vi "State Machine.vi"() -> ()   [LabVIEW 2014]
uses:
  Enum.ctl
panel:
  in  "STOP":bool
  in  "Executer le processus 2":bool
  in  "Executer le processus 1":bool
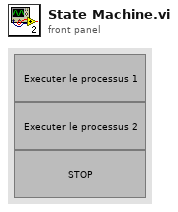
[diagram p1: front panel]
types:
  T1 = typedef "Enum.ctl" = enum16{"Inactif", "Processus 1", "Processus 2", "Arret"}
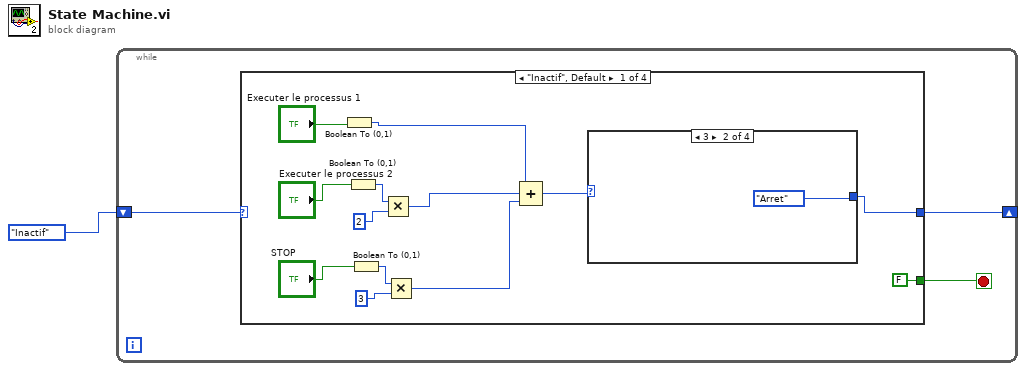
[diagram p0: block diagram]
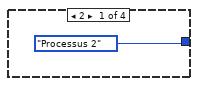
[diagram p2: hidden frame]
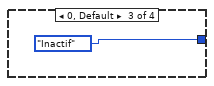
[diagram p3: hidden frame]
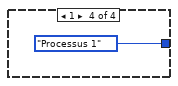
[diagram p4: hidden frame]
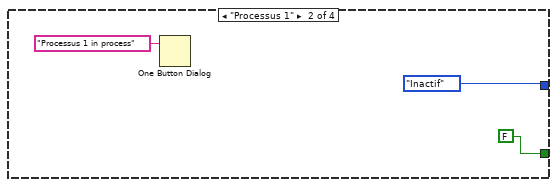
[diagram p5: hidden frame]
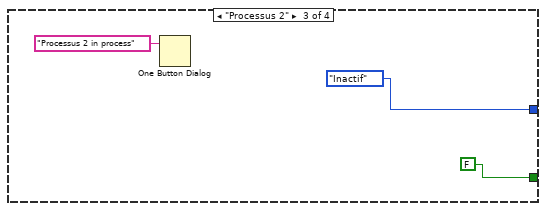
[diagram p6: hidden frame]
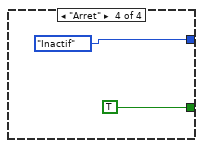
[diagram p7: hidden frame]
diagram:
  n1 = while {
    shift-right: [w3] -> _
    shift-left: Enum."Inactif" -> [w4]
    stop <- w2 stop-if-true
    n2 = case shown="\"Inactif\", Default" w4 {
      tunnel: [w6 Enum."Inactif" Enum."Inactif" Enum."Inactif"] -> w3
      tunnel: [FALSE FALSE FALSE TRUE] -> w2
      frame "Inactif", Default {
        n3 = Boolean To (0,1)(Boolean="Executer le processus 1") -> (0, 1=w12:i16)
        n4 = Boolean To (0,1)(Boolean="Executer le processus 2") -> (0, 1=w15:i16)
        n5 = Boolean To (0,1)(Boolean="STOP") -> (0, 1=w14:i16)
        n6 = Multiply(x=w15, y=2) -> (x*y=w11:i32)
        n7 = Multiply(x=w14, y=3) -> (x*y=w7:i32)
        n8 = Compound Arithmetic op=ADD(w12, w11, w7) -> (w8:i32)
        n9 = case shown="3" w8 {
          tunnel: [Enum."Processus 2" Enum."Arret" Enum."Inactif" Enum."Processus 1"] -> w6
          frame 2 {
          }
          frame 3 {
          }
          frame 0, Default {
          }
          frame 1 {
          }
        }
      }
      frame "Processus 1" {
        n10 = One Button Dialog(message="Processus 1 in process") -> ()  [unwired: 1 in, 1 out]
      }
      frame "Processus 2" {
        n11 = One Button Dialog(message="Processus 2 in process") -> ()  [unwired: 1 in, 1 out]
      }
      frame "Arret" {
      }
    }
  }
